vi "服务端侦听.vi"(0 "MainPage 输入":refnum<class "MainPage.lvclass">) -> ()   [LabVIEW 2019, in "MainPage.lvlib" / "MainPage.lvclass"]
uses:
  MainPage.lvclass
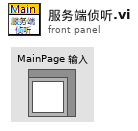
[diagram p1: front panel]
types:
  T1 = typedef "MainPage.lvlib/MainPage.lvclass/DataRef_通讯接口.ctl" = cluster{"连接方式":enum16{"网口(客服端)", "网口(服务端)", "串口"}, "VISA串口名称":refnum<visa-resource-name>, "服务端识别":cluster{"本机IP":string, "本机端口":u16, "当前目标":string, "服务端侦听ID":refnum<k5>}, "客服端识别":cluster{"客P-主IP:Port":string}, "客服端记录":map{string, refnum<k5>}, "服务端接口记录":map{string, refnum<k5>}}
  T2 = cluster{"寄存器模拟":u16[], "串口正常？":bool, "报文信息记录":string[][]}
  T3 = enum16{"ini", "增加记录", "读取记录", "更改寄存器值", "更改接口状态", "更改报文信息", "增加报文信息"}
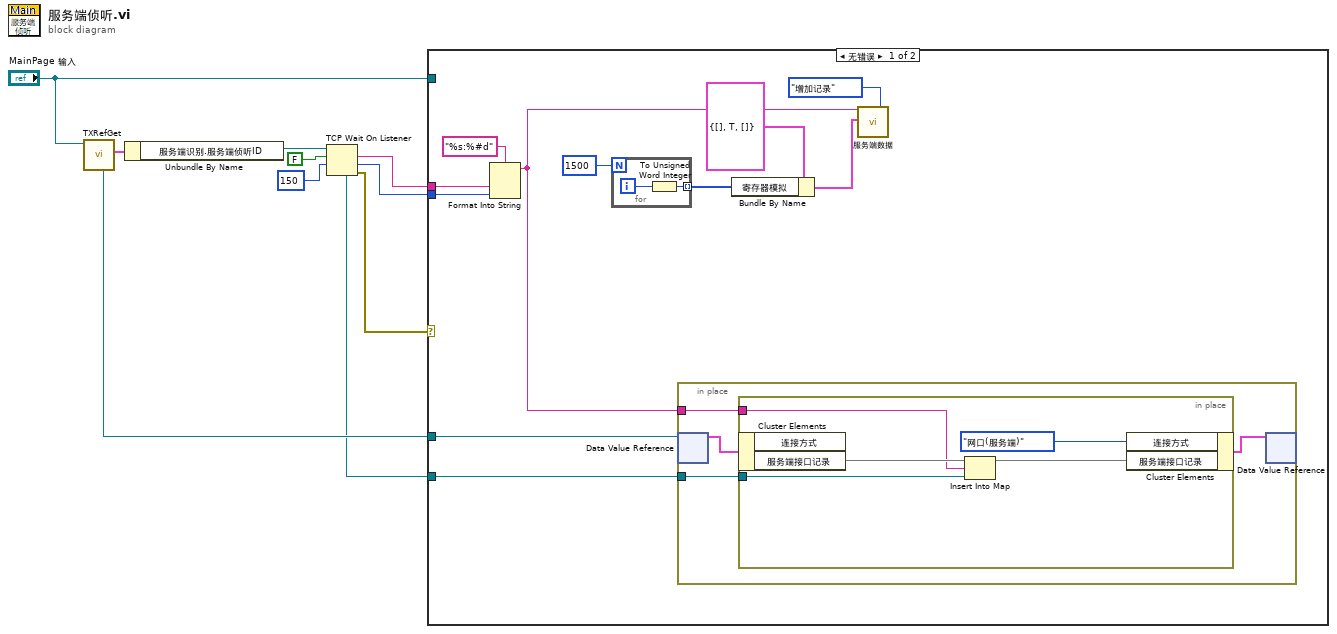
[diagram p0: block diagram]
diagram:
  n1 = call-dynamic "TXRefGet.vi"("MainPage 输入"="MainPage 输入") -> ("通讯接口数据"=w10:T1, "引用"=w4:refnum<data-value>)  [unwired: 6 in, 3 out]
  n2 = Unbundle By Name(w10) -> ("服务端识别.服务端侦听ID"=w9:refnum<k5>)
  n3 = TCP Wait On Listener(9:150 ("超时毫秒（一直等待:-1）"), 10:FALSE ("解析远程地址(T)"), 11:w9) -> (0:w5:errorcluster, 1:w1:u16, 2:w2:string, 4:w3:refnum<k5>)  [unwired: 1 in, 1 out]
  n4 = case shown="无错误" w5 {
    tunnel: "MainPage 输入" -> [_ _]
    tunnel: w4 -> [w20 _]
    tunnel: w3 -> [w19 _]
    tunnel: w2 -> [w17 _]
    tunnel: w1 -> [w16 _]
    frame No Error {
      n5 = Format Into String(format string="%s:%#d" ("格式字符串"), w17, w16) -> (resulting string=w14:string)  [unwired: 2 in, 1 out]
      n6 = for {
        N: 1500 -> [_]
        tunnel: [w31] -> w11 mode=indexing
        i -> [w32]
        n7 = To Unsigned Word Integer(number=w32) -> (unsigned 16bit integer=w31:u16)
      }
      n8 = in-place {
        in-place-border: w14 -> [w23]
        in-place-border: w19 -> [w22]
        n9 = in-place-dvr #1(w20) -> (w25:T1)  [unwired: 1 out]
        n10 = in-place {
          in-place-border: w23 -> [w28]
          in-place-border: w22 -> [w27]
          n11 = in-place-cluster #2(w25) -> ("服务端接口记录"=w30:map{string, refnum<k5>})  [unwired: 1 out]
          n12 = Insert Into Map(map in=w30, key=w28, value=w27) -> (map out=w29:map{string, refnum<k5>})  [unwired: 2 out]
          n13 = in-place-cluster #2("连接方式"=enum16{"网口(客服端)", "网口(服务端)", "串口"}."网口(服务端)", "服务端接口记录"=w29) -> (w24:T1)
        }
        n14 = in-place-dvr #1(w24) -> ()  [unwired: 2 out]
      }
      n15 = Bundle By Name(cluster=T2 {"寄存器模拟"=[], "串口正常？"=TRUE, "报文信息记录"=[]} ("值"), "寄存器模拟"=w11) -> (w12:T2)
      n16 = call "服务端数据.vi"("IP-Port"=w14, "数据输入"=w12, "枚举"=T3."增加记录") -> ()  [unwired: 15 in, 2 out]
    }
    frame Error {
    }
  }
